vi "ForceUpdate.vi"(1 "Set":bool) -> (15 "Force":bool)   [LabVIEW 2016, in "Grid.lvclass"]
uses:
  <resource>/Framework/Providers/Open_GDS/UML/Grid_class/Grid.lvclass
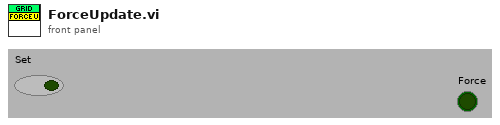
[diagram p1: front panel]
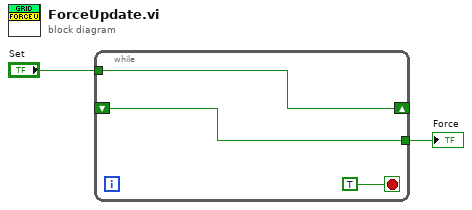
[diagram p0: block diagram]
diagram:
  n1 = while {
    shift-right: [w5] -> _
    shift-left: _ -> [w4]
    tunnel: "Set" -> [w5]
    tunnel: [w4] -> w1
    stop <- TRUE stop-if-true
  }
  "Force" <- w1
